vi "interface.vi"(8 "error in (no error)":errorcluster) -> (0 "error out":errorcluster)   [LabVIEW 2020]
uses:
  Control 1.ctl
  <vilib>/Utility/sysdir.llb/System Directory Type.ctl
  <vilib>/Utility/miscctls.llb/LVRowAndColumnUnsignedTypeDef.ctl
  <vilib>/Utility/config.llb/Write Key (String).vi
  <vilib>/Utility/config.llb/Write Key (Path).vi
  <vilib>/Utility/config.llb/Read Key (String).vi
  <vilib>/Utility/config.llb/Read Key (Path).vi
  _Common_Lib/UI/Window Msg/Window Msg.lvclass
  <vilib>/WebDAVClient/NI_WebDAV.lvlib
  <vilib>/Utility/config.llb/NI_LVConfig.lvlib
panel:
  in  "Delete cRIO folder(s) after download":bool
  in  "Download folder":path
  in  "Search directories":bool
  in  "cRIO IP address":string="172.22.11.2"
  in  "Open folder after download":bool
  in  "Folder path":string="/home/lvuser"
  in  "Start retrieving directories":bool
  in  "Directories list":i32[](listbox)
  # "Please select all folders that have to be retrieved from cRIO"
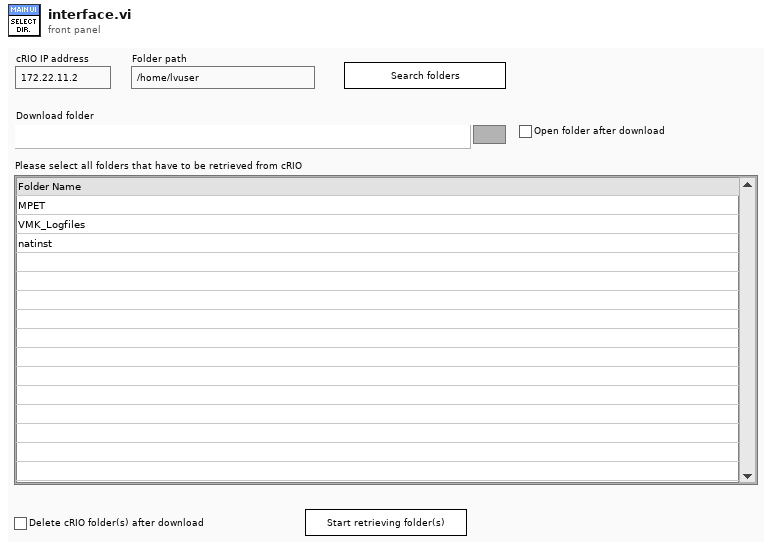
[diagram p1: front panel]
types:
  T1 = typedef "System Directory Type.ctl" = i32
  T2 = typedef "Control 1.ctl" = enum16{"READ CRIO FOLDERS", "DOWNLOAD", "IDLE", "READ SETTINGS", "ERROR", "EXIT"}
  T3 = typedef "LVRowAndColumnUnsignedTypeDef.ctl" = cluster{"Row":u32, "Column":u32}
  T4 = enum16{"INIT", "LOAD", "IDLE", "GRAPH", "ERROR", "EXIT"}
  T5 = typedef "NI_WebDAV.lvlib/SessionHandle.ctl" = refnum<k1>
  T6 = typedef "NI_WebDAV.lvlib/FileInfo.ctl" = cluster{"type":string, "size":u64, "last modification":timestamp, "display name":string, "uri":string}
  T7 = typedef "NI_LVConfig.lvlib/Config Data RefNum.ctl" = refnum<k1>
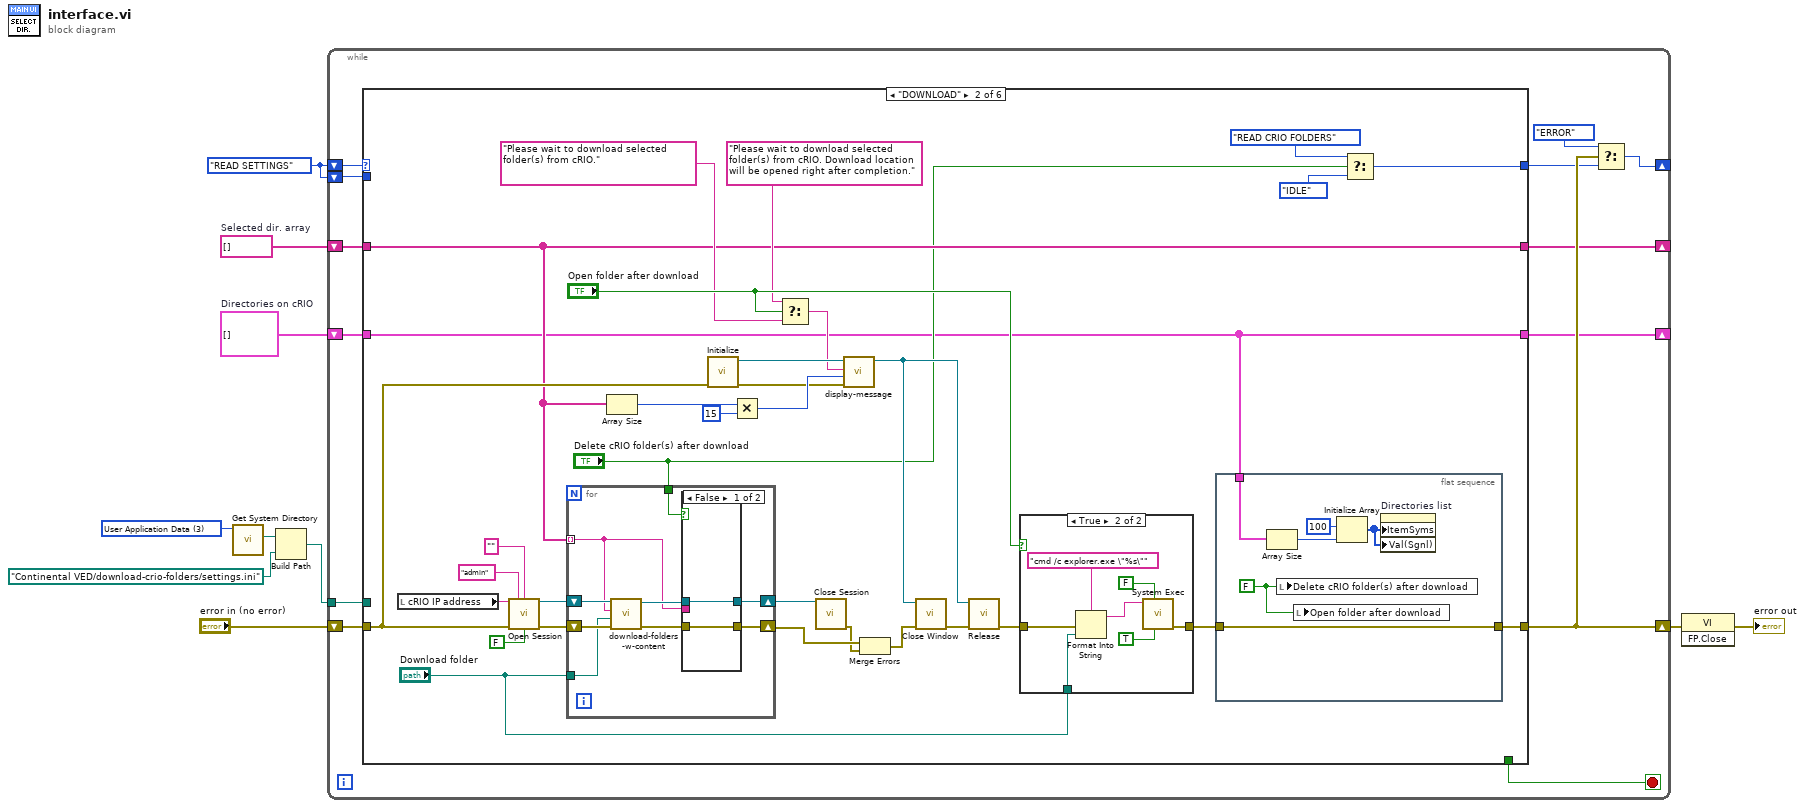
[diagram p0: block diagram]
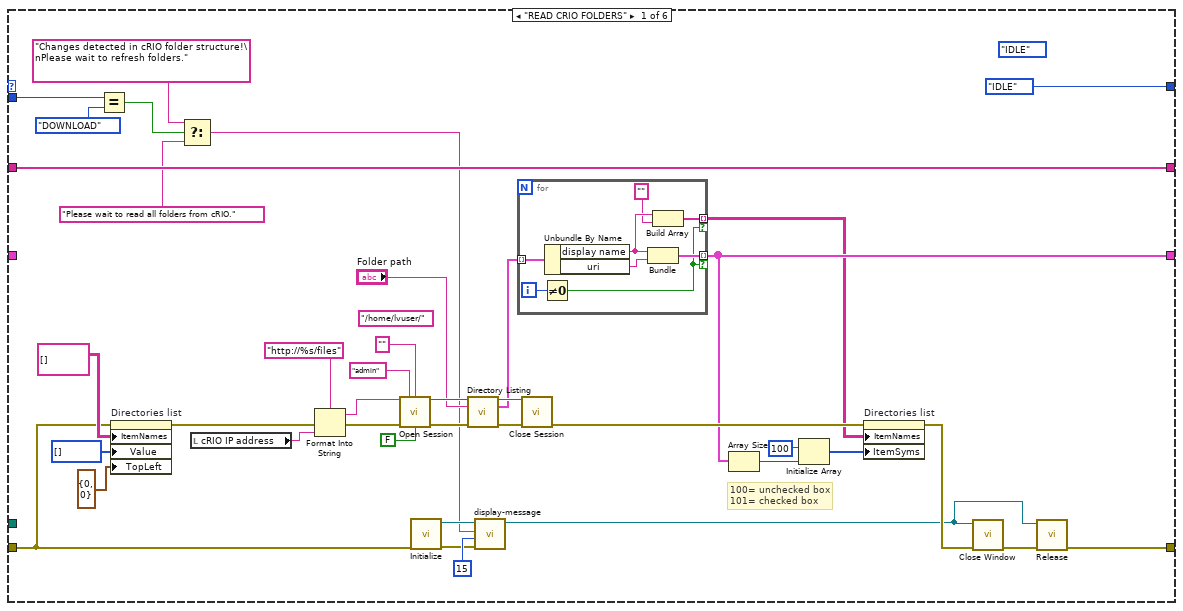
[diagram p2: hidden frame]
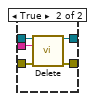
[diagram p4: hidden frame]
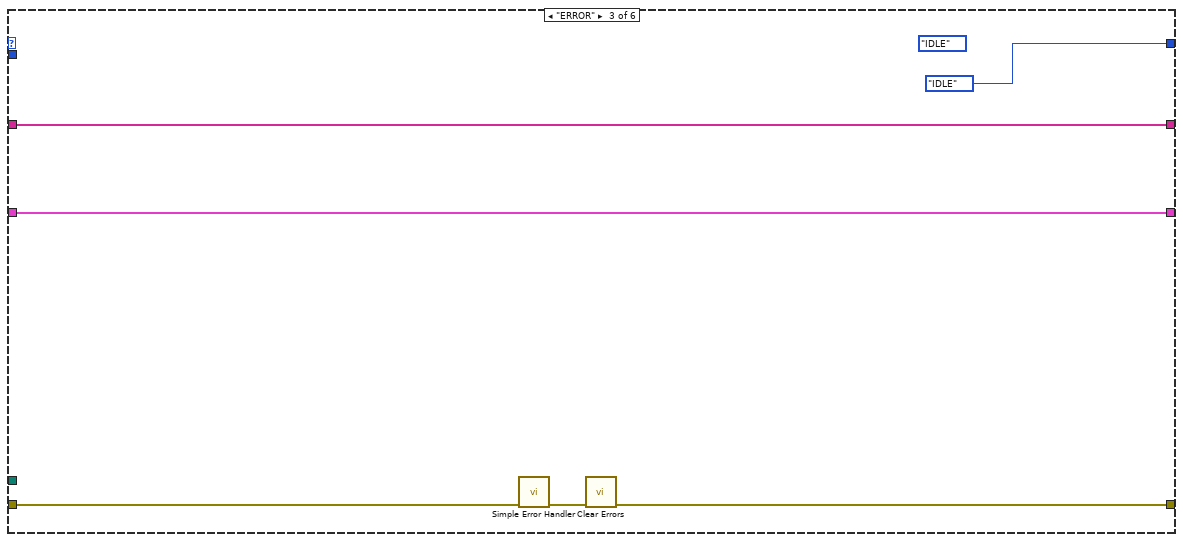
[diagram p5: hidden frame]
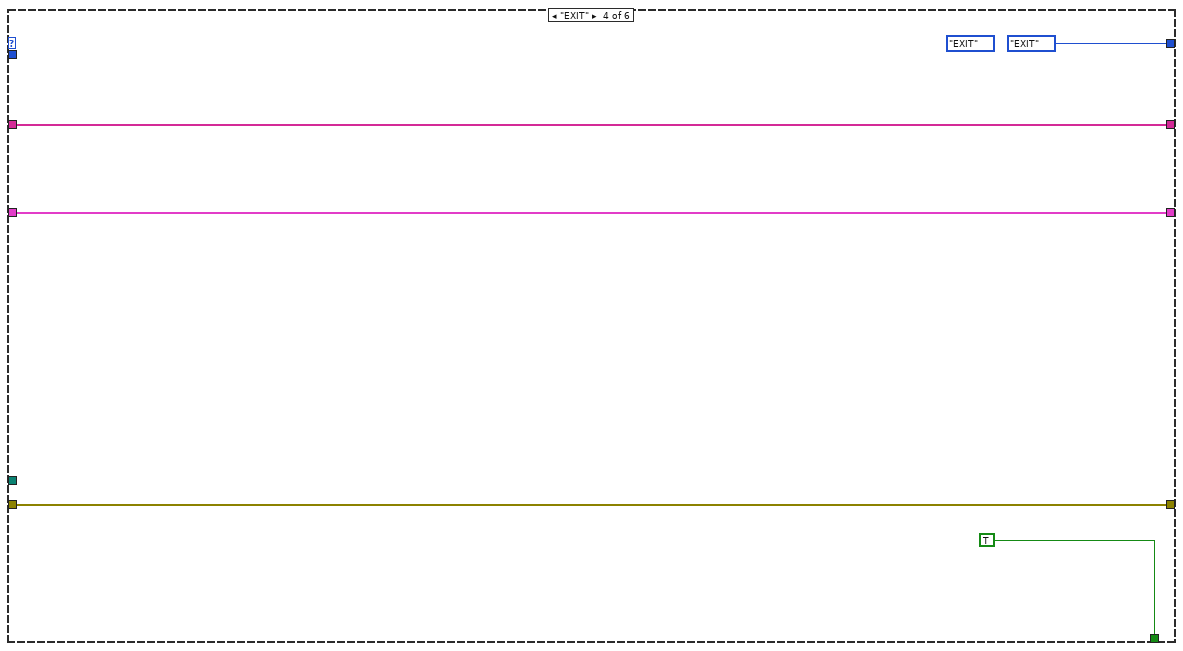
[diagram p6: hidden frame]
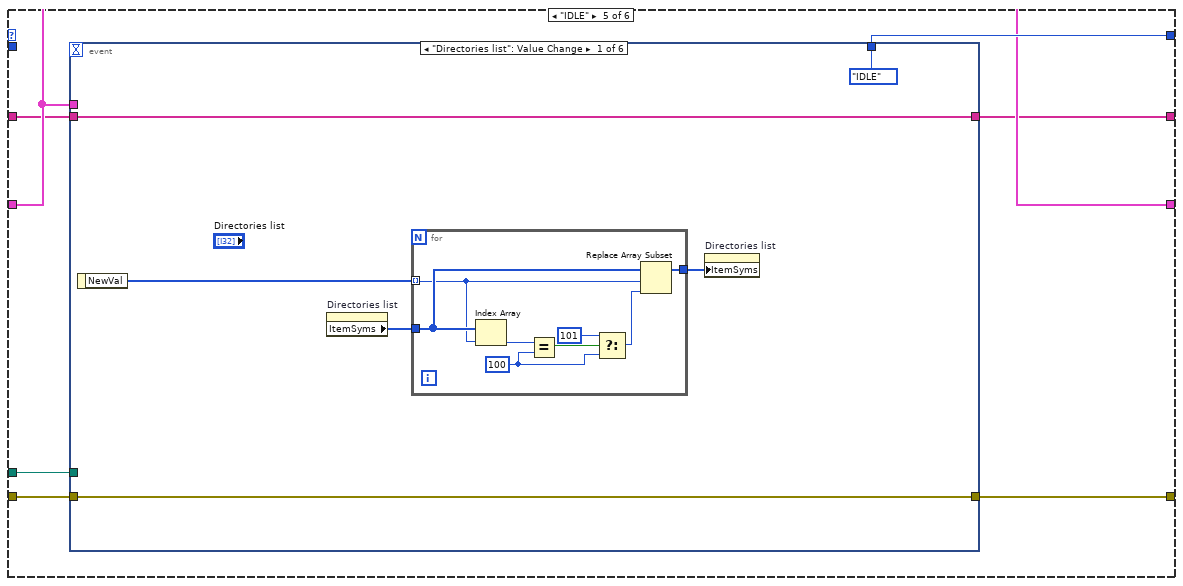
[diagram p7: hidden frame]
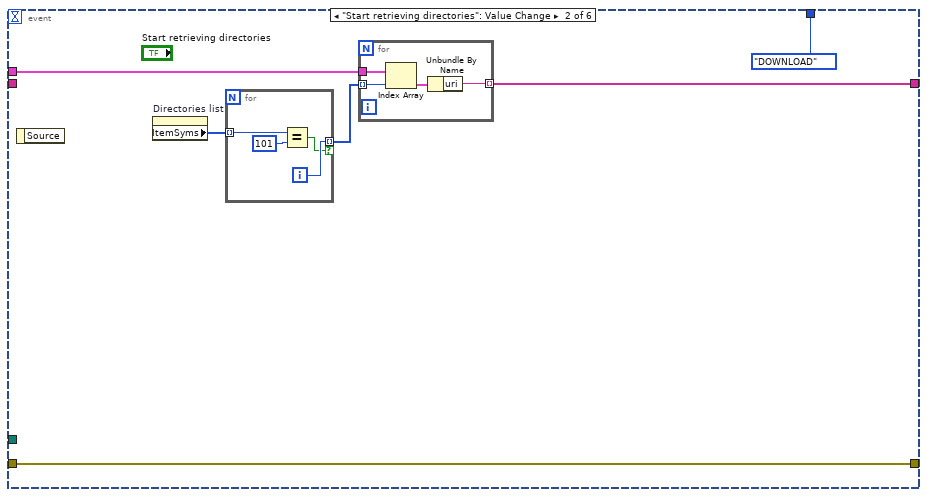
[diagram p8: hidden frame]
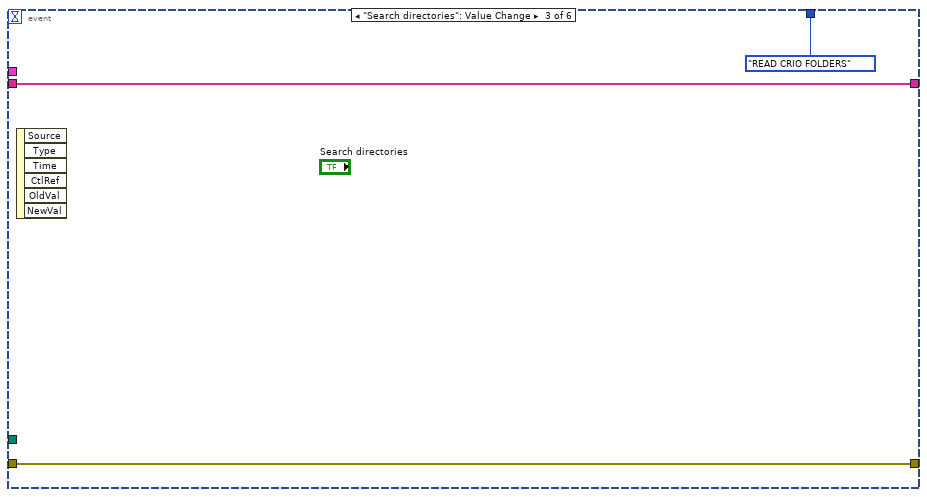
[diagram p9: hidden frame]
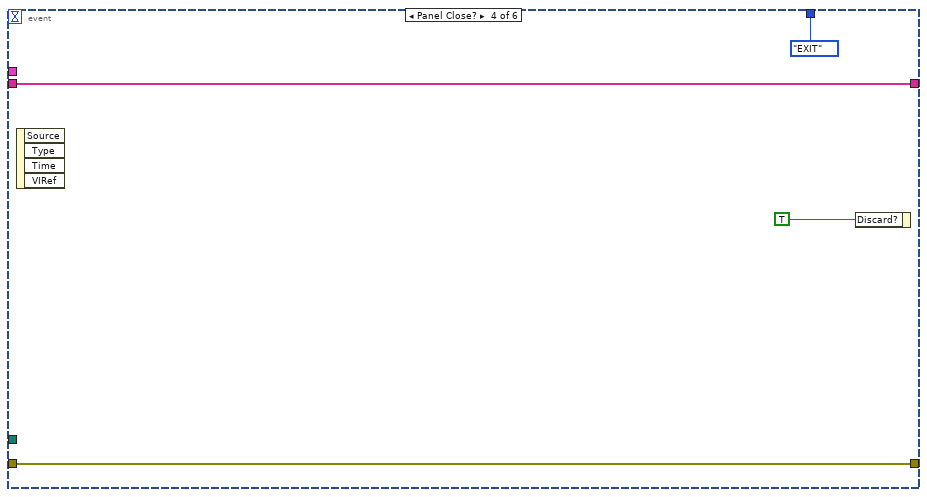
[diagram p10: hidden frame]
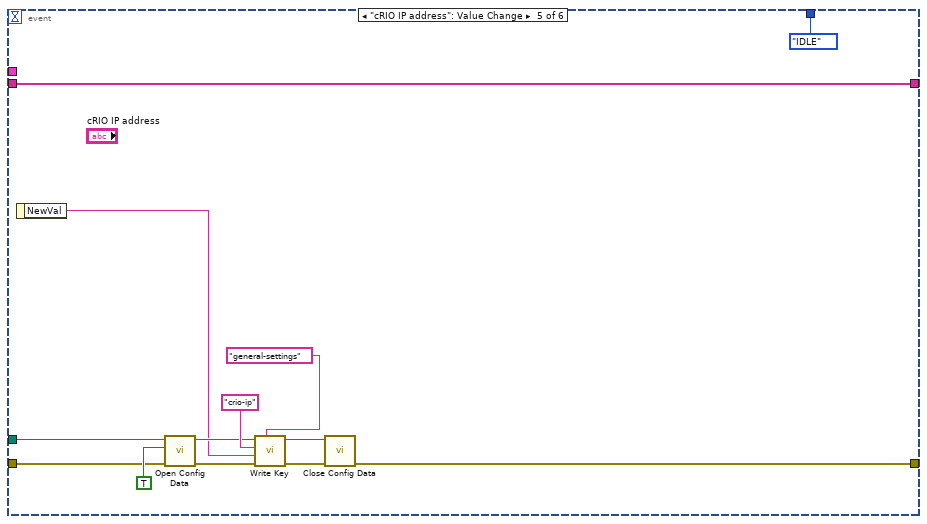
[diagram p11: hidden frame]
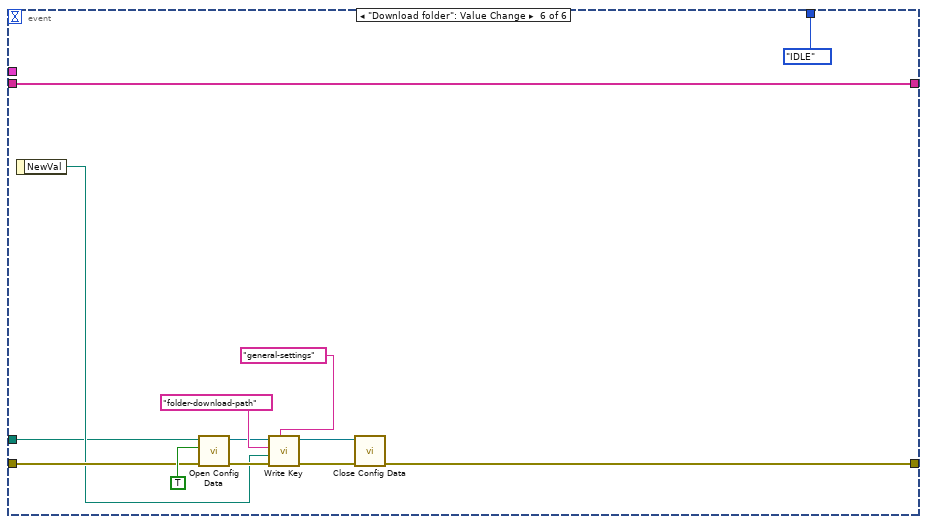
[diagram p12: hidden frame]
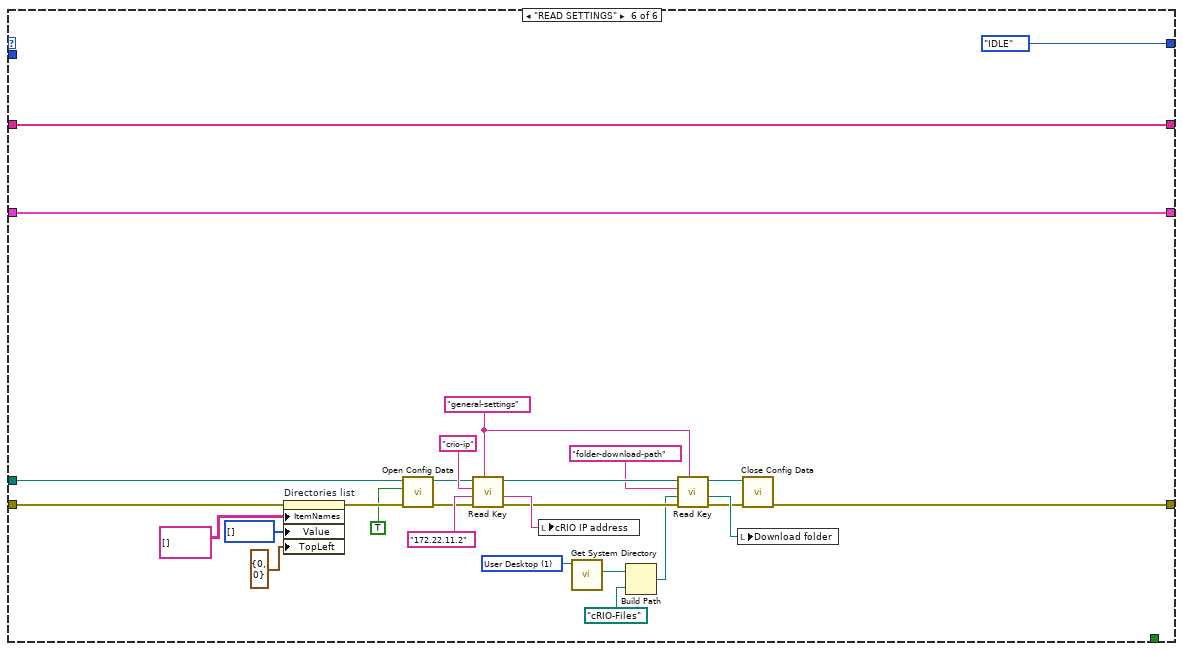
[diagram p13: hidden frame]
diagram:
  w5 = T1 3 items=["User Home"=0, "User Desktop"=1, "User Documents"=2, "User Application Data"=3, "User Preferences"=4, "User Temporary"=5, "Public Documents"=6, "Public Application Data"=7, "Public Preferences"=8, "Public Cache"=13, "System Core Libraries"=9, "System Installed Libraries"=10, "Application Files"=11, "Boot Volume Root"=12] ("system directory type")
  w1 = Control_1."READ SETTINGS" ("Motor Logger Viewer Action")
  w9 = string[] []  # Selected dir. array
  w10 = cluster{"display name":string, "uri":string}[] []  # Directories on cRIO
  n1 = call <vilib>:"Get System Directory.vi"("system directory type"=w5) -> ("system directory"=w4:path)  [unwired: 10 in]
  n2 = Build Path(base path=w4, name or relative path=path "Continental VED/download-crio-folders/settings.ini" ("configuration file path")) -> (appended path=w2:path)
  n3 = while {
    shift-right: [w20] -> w8
    shift-left: "error in (no error)" -> [w22]
    shift-right: [w18] -> _
    shift-left: w1 -> [w23]
    shift-right: [w17] -> _
    shift-left: w10 -> [w16]
    shift-right: [w15] -> _
    shift-left: w9 -> [w14]
    tunnel: w2 -> [w13]
    shift-left: w1 -> [w11]
    stop <- w21 stop-if-true
    n4 = case shown="\"DOWNLOAD\"" w23 {
      tunnel: w22 -> [w48 w93 w137 w142 w144 w214]
      tunnel: [w38 w76 w136 w142 w145 w215] -> w20
      tunnel: [_ _ _ TRUE _ _] -> w21
      tunnel: [Control_1."IDLE" ("Motor Logger Viewer Action") w72 Control_1."IDLE" ("Motor Logger Viewer Action") Control_1."EXIT" ("Motor Logger Viewer Action") w150 Control_1."IDLE" ("Motor Logger Viewer Action")] -> w19
      tunnel: [w42 w71 w135 w141 w149 w238] -> w17
      tunnel: w16 -> [_ w71 w135 w141 w149 w238]
      tunnel: [w40 w83 w134 w140 w148 w237] -> w15
      tunnel: w14 -> [w40 w83 w134 w140 w147 w237]
      tunnel: w13 -> [_ _ _ _ w146 w213]
      tunnel: w11 -> [w30 _ _ _ _ _]
      frame "READ CRIO FOLDERS" {
        (unwired) T4."IDLE" ("Motor Logger Viewer Action")
        (unwired) "/home/lvuser/" ("relative uri")
        # "100= unchecked box\n101= checked box"
        n5 = Equal?(x=w30, y=Control_1."DOWNLOAD") -> (x = y?=w28:bool)
        n6 = property on="Directories list" class="MCListbox (strict)"(error in=w48, "ItemNames"=string[][] [] ("Item Names"), "Value"=i32[] [] ("Directories list"), "TopLeft"=T3 {"Row"=0, "Column"=0} ("Top Left Visible Cell")) -> (error out=w36:errorcluster)  [unwired: 1 in, 1 out]
        n7 = Select(t="Changes detected in cRIO folder structure!\nPlease wait to refresh folders.", s=w28, f="Please wait to read all folders from cRIO." ("Message")) -> (s? t:f=w25:string)
        n8 = local read "cRIO IP address"() -> (w32:string)
        n9 = Format Into String(format string="http://%s/files", error in=w36, w32) -> (resulting string=w56:string, error out=w53:errorcluster)  [unwired: 1 in]
        n10 = call <vilib>:"Open Session.vi"("host uri prefix"=w56, "username"="admin", "password"="", "error in (no error)"=w53, "verify server?"=FALSE) -> ("session handle out"=w62:T5, "error out"=w61:errorcluster)  [unwired: 9 in]
        n11 = call "Initialize.vi"("error in (no error)"=w48) -> ("error out"=w33:errorcluster, "Window Msg out"=w52:refnum<class "Window Msg.lvclass">)  [unwired: 9 in]
        n12 = call <vilib>:"Directory Listing.vi"("session handle"=w62, "relative uri"="Folder path", "error in (no error)"=w61) -> ("session handle out"=w54:T5, "directory list"=w50:T6[], "error out"=w55:errorcluster)  [unwired: 9 in, 1 out]
        n13 = call "display-message.vi"("error in (no error)"=w33, "Time to wait (x*100ms)"=15 ("Time to wait (*500ms)"), "Message"=w25, "Window Msg in"=w52) -> ("Window Msg out"=w35:refnum<class "Window Msg.lvclass">)  [unwired: 6 in, 1 out]
        n14 = for {
          tunnel: w50 -> [w70] mode=indexing
          tunnel: [w68] -> w42 mode=indexing if=w63
          tunnel: [w64] -> w24 mode=indexing if=w63
          i -> [w67]
          n15 = Not Equal To 0?(x=w67) -> (x != 0?=w63:bool)
          n16 = Unbundle By Name(w70) -> ("display name"=w66:string, "uri"=w69:string)
          n17 = Bundle("display name"=w66, "uri"=w69) -> (w68:cluster{"display name":string, "uri":string})  [unwired: 1 in]
          n18 = Build Array(w66, "" ("display name")) -> (w64:string[])
        }
        n19 = call <vilib>:"Close Session.vi"("session handle"=w54, "error in (no error)"=w55) -> ("error out"=w45:errorcluster)  [unwired: 13 in]
        n20 = Array Size(array=w42) -> (size(s)=w43:i32)
        n21 = Initialize Array(100, w43) -> (w41:i32[])
        n22 = property on="Directories list" class="MCListbox (strict)"(error in=w45, "ItemNames"=w24, "ItemSyms"=w41) -> (error out=w39:errorcluster)  [unwired: 1 in, 1 out]
        n23 = call "Close Window.vi"("error in (no error)"=w39, "Window Msg in"=w35) -> ("error out"=w51:errorcluster)  [unwired: 9 in]
        n24 = call "Release.vi"("error in (no error)"=w51, "Window Msg in"=w35) -> ("error out"=w38:errorcluster)  [unwired: 9 in]
      }
      frame "DOWNLOAD" {
        n25 = local read "cRIO IP address"() -> (w99:string)
        n26 = call <vilib>:"Open Session.vi"("host uri prefix"=w99, "username"="admin", "password"="", "error in (no error)"=w93, "verify server?"=FALSE) -> ("session handle out"=w97:T5, "error out"=w98:errorcluster)  [unwired: 9 in]
        n27 = for {
          shift-right: [w125] -> w96
          shift-left: w98 -> [w121]
          tunnel: "Download folder" -> [w120]
          tunnel: "Delete cRIO folder(s) after download" -> [w124]
          shift-right: [w123] -> w84
          shift-left: w97 -> [w122]
          tunnel: w83 -> [w117] mode=indexing
          n28 = call "download-folders-w-content.vi"("error in"=w121, "download folder"=w120, "relative uri"=w117, "session handle in"=w122) -> ("error out"=w119:errorcluster, "session handle out"=w118:T5)  [unwired: 6 in]
          n29 = case shown="False" w124 {
            tunnel: w117 -> [_ w132]
            tunnel: w119 -> [w127 w131]
            tunnel: [w127 w130] -> w125
            tunnel: w118 -> [w126 w129]
            tunnel: [w126 w128] -> w123
            frame False {
            }
            frame True {
              n30 = call <vilib>:"Delete.vi"("session handle"=w129, "relative uri"=w132, "error in (no error)"=w131) -> ("session handle out"=w128:T5, "error out"=w130:errorcluster)  [unwired: 11 in]
            }
          }
        }
        n31 = Array Size(array=w83) -> (size(s)=w92:i32)
        n32 = call "Initialize.vi"("error in (no error)"=w93) -> ("error out"=w79:errorcluster, "Window Msg out"=w82:refnum<class "Window Msg.lvclass">)  [unwired: 9 in]
        n33 = Multiply(x=w92, y=15) -> (x*y=w80:i32)
        n34 = Select(t="Please wait to download selected folder(s) from cRIO. Download location will be opened right after completion." ("Message"), s="Open folder after download", f="Please wait to download selected folder(s) from cRIO." ("Message")) -> (s? t:f=w81:string)
        n35 = call <vilib>:"Close Session.vi"("session handle"=w84) -> ("error out"=w95:errorcluster)  [unwired: 14 in]
        n36 = call "display-message.vi"("error in (no error)"=w79, "Time to wait (x*100ms)"=w80, "Message"=w81, "Window Msg in"=w82) -> ("Window Msg out"=w78:refnum<class "Window Msg.lvclass">)  [unwired: 6 in, 1 out]
        n37 = Merge Errors(w96, w95) -> (w90:errorcluster)
        n38 = call "Close Window.vi"("error in (no error)"=w90, "Window Msg in"=w78) -> ("error out"=w94:errorcluster)  [unwired: 9 in]
        n39 = call "Release.vi"("error in (no error)"=w94, "Window Msg in"=w78) -> ("error out"=w89:errorcluster)  [unwired: 9 in]
        n40 = case shown="True" "Open folder after download" {
          tunnel: "Download folder" -> [_ w112]
          tunnel: [w109 w111] -> w77
          tunnel: w89 -> [w109 w110]
          frame False {
          }
          frame True {
            n41 = Format Into String(format string="cmd /c explorer.exe \"%s\"" ("command line"), error in=w110, w112) -> (resulting string=w115:string)  [unwired: 1 in, 1 out]
            n42 = call <vilib>:"System Exec.vi"("run minimized? (F)"=TRUE, "wait until completion? (T)"=FALSE, "command line"=w115) -> ("error out"=w111:errorcluster)  [unwired: 5 in, 3 out]
          }
        }
        n43 = flat-sequence {
          tunnel: w77 -> [w108]
          tunnel: [w108] -> w76
          tunnel: w71 -> [w104]
          frame #0 {
            w107 = FALSE ("Delete cRIO folder(s) after download")
            n44 = Array Size(array=w104) -> (size(s)=w106:i32)
            n45 = local write "Delete cRIO folder(s) after download"(w107) -> ()
            n46 = local write "Open folder after download"(w107) -> ()
            n47 = Initialize Array(100, w106) -> (w103:i32[])
            n48 = property on="Directories list" class="MCListbox (strict)"("ItemSyms"=w103, "Val(Sgnl)"=w103) -> ()  [unwired: 2 in, 2 out]
          }
        }
        n49 = Select(t=Control_1."READ CRIO FOLDERS" ("Motor Logger Viewer Action"), s="Delete cRIO folder(s) after download", f=Control_1."IDLE") -> (s? t:f=w72:T2)
      }
      frame "ERROR" {
        (unwired) T4."IDLE" ("Motor Logger Viewer Action")
        n50 = call <vilib>:"Simple Error Handler.vi"("error in (no error)"=w137) -> ("error out"=w138:errorcluster)  [unwired: 4 in, 4 out]
        n51 = call <vilib>:"Clear Errors.vi"("error in (no error)"=w138) -> ("error out"=w136:errorcluster)  [unwired: 5 in, 1 out]
      }
      frame "EXIT" {
        (unwired) T4."EXIT" ("Motor Logger Viewer Action")
      }
      frame "IDLE" {
        n52 = event shown="[0] \"Directories list\": Value Change" {
          selector: _ -> [_ _ _ _ _ _]
          dyn-events: _ -> [_ _ _ _ _ _]
          timeout: _ -> [_ _ _ _ _ _]
          tunnel: [Control_1."IDLE" ("Motor Logger Viewer Action") Control_1."DOWNLOAD" ("Motor Logger Viewer Action") Control_1."READ CRIO FOLDERS" ("Motor Logger Viewer Action") Control_1."EXIT" ("Motor Logger Viewer Action") Control_1."IDLE" ("Motor Logger Viewer Action") Control_1."IDLE" ("Motor Logger Viewer Action")] -> w150
          tunnel: w149 -> [_ w169 _ _ _ _]
          tunnel: [w153 w167 w181 w184 w198 w211] -> w148
          tunnel: w147 -> [w153 _ w181 w184 w198 w211]
          tunnel: w146 -> [_ _ _ _ w193 w200]
          tunnel: w144 -> [w152 w166 w180 w183 w192 w203]
          tunnel: [w152 w166 w180 w183 w191 w202] -> w145
          event "Directories list": Value Change {
            n53 = event-data() -> ("NewVal"=w156:i32[])  [unwired: 1 in]
            n54 = property on="Directories list" class="MCListbox (strict)"() -> ("ItemSyms"=w155:i32[])  [unwired: 2 in, 2 out]
            n55 = for {
              tunnel: w156 -> [w158] mode=indexing
              tunnel: w155 -> [w160]
              tunnel: [w157] -> w154
              w162 = 100 ("y")
              n56 = Index Array(array=w160, index=w158) -> (element=w164:i32)
              n57 = Equal?(x=w164, y=w162) -> (x = y?=w163:bool)
              n58 = Select(t=101, s=w163, f=w162) -> (s? t:f=w159:i32)
              n59 = Replace Array Subset(array=w160, new element=w159, index=w158) -> (w157:i32[])
            }
            n60 = property on="Directories list" class="MCListbox (strict)"("ItemSyms"=w154) -> ()  [unwired: 2 in, 2 out]
          }
          event "Start retrieving directories": Value Change {
            n61 = event-data() -> ()  [unwired: 1 in, 1 out]
            n62 = property on="Directories list" class="MCListbox (strict)"() -> ("ItemSyms"=w170:i32[])  [unwired: 2 in, 2 out]
            n63 = for {
              tunnel: w170 -> [w178] mode=indexing
              tunnel: [w176] -> w168 mode=indexing if=w175
              i -> [w176]
              n64 = Equal?(x=w178, y=101) -> (x = y?=w175:bool)
            }
            n65 = for {
              tunnel: w169 -> [w174]
              tunnel: w168 -> [w173] mode=indexing
              tunnel: [w171] -> w167 mode=indexing
              n66 = Index Array(array=w174, index=w173) -> (element=w172:cluster{"display name":string, "uri":string})
              n67 = Unbundle By Name(w172) -> ("uri"=w171:string)
            }
          }
          event "Search directories": Value Change {
            n68 = event-data() -> ()  [unwired: 1 in, 6 out]
          }
          event Panel Close? {
            n69 = event-data() -> ()  [unwired: 1 in, 4 out]
            n70 = event-data("Discard?"=TRUE) -> ()  [unwired: 1 in, 1 out]
          }
          event "cRIO IP address": Value Change {
            n71 = event-data() -> ("NewVal"=w187:string)  [unwired: 1 in]
            n72 = call <vilib>:"Open Config Data.vi"("error in (no error)"=w192, "create file if necessary (T)"=TRUE, "configuration file path"=w193) -> ("error out"=w196:errorcluster, "refnum"=w195:T7)  [unwired: 6 in, 1 out]
            n73 = call-poly <vilib>:"Write Key.vi"("section"="general-settings", "error in (no error)"=w196, "value"=w187, "key"="crio-ip", "refnum"=w195) -> ("error out"=w189:errorcluster, "refnum out"=w190:T7)  [unwired: 4 in, 1 out]
            n74 = call <vilib>:"Close Config Data.vi"("error in (no error)"=w189, "refnum"=w190) -> ("error out"=w191:errorcluster)  [unwired: 8 in, 1 out]
          }
          event "Download folder": Value Change {
            n75 = event-data() -> ("NewVal"=w201:path)  [unwired: 1 in]
            n76 = call <vilib>:"Open Config Data.vi"("error in (no error)"=w203, "create file if necessary (T)"=TRUE, "configuration file path"=w200) -> ("error out"=w209:errorcluster, "refnum"=w208:T7)  [unwired: 6 in, 1 out]
            n77 = call-poly <vilib>:"Write Key.vi"("section"="general-settings", "error in (no error)"=w209, "value"=w201, "key"="folder-download-path", "refnum"=w208) -> ("error out"=w205:errorcluster, "refnum out"=w206:T7)  [unwired: 4 in, 1 out]
            n78 = call <vilib>:"Close Config Data.vi"("error in (no error)"=w205, "refnum"=w206) -> ("error out"=w202:errorcluster)  [unwired: 8 in, 1 out]
          }
        }
      }
      frame "READ SETTINGS" {
        w233 = "general-settings" ("section")
        w216 = T1 1 items=["User Home"=0, "User Desktop"=1, "User Documents"=2, "User Application Data"=3, "User Preferences"=4, "User Temporary"=5, "Public Documents"=6, "Public Application Data"=7, "Public Preferences"=8, "Public Cache"=13, "System Core Libraries"=9, "System Installed Libraries"=10, "Application Files"=11, "Boot Volume Root"=12] ("system directory type")
        n79 = property on="Directories list" class="MCListbox (strict)"(error in=w214, "ItemNames"=string[][] [] ("Item Names"), "Value"=i32[] [] ("Directories list"), "TopLeft"=T3 {"Row"=0, "Column"=0} ("Top Left Visible Cell")) -> (error out=w231:errorcluster)  [unwired: 1 in, 1 out]
        n80 = call <vilib>:"Open Config Data.vi"("error in (no error)"=w231, "create file if necessary (T)"=TRUE, "configuration file path"=w213) -> ("error out"=w228:errorcluster, "refnum"=w227:T7)  [unwired: 6 in, 1 out]
        n81 = call-poly <vilib>:"Read Key.vi"("section"=w233, "error in (no error)"=w228, "default value"="172.22.11.2", "key"="crio-ip", "refnum"=w227) -> ("error out"=w229:errorcluster, "value"=w232:string, "refnum out"=w230:T7)  [unwired: 3 in, 1 out]
        n82 = local write "cRIO IP address"(w232) -> ()
        n83 = call <vilib>:"Get System Directory.vi"("system directory type"=w216) -> ("system directory"=w217:path)  [unwired: 10 in]
        n84 = Build Path(base path=w217, name or relative path=path "cRIO-Files" ("base path")) -> (appended path=w222:path)
        n85 = call-poly <vilib>:"Read Key.vi"("section"=w233, "error in (no error)"=w229, "default value"=w222, "key"="folder-download-path", "refnum"=w230) -> ("error out"=w224:errorcluster, "value"=w235:path, "refnum out"=w225:T7)  [unwired: 3 in, 1 out]
        n86 = local write "Download folder"(w235) -> ()
        n87 = call <vilib>:"Close Config Data.vi"("error in (no error)"=w224, "refnum"=w225) -> ("error out"=w215:errorcluster)  [unwired: 8 in, 1 out]
      }
    }
    n88 = Select(t=Control_1."ERROR" ("Motor Logger Viewer Action"), s=w20, f=w19) -> (s? t:f=w18:T2)
  }
  n89 = invoke class="VI" method="FP.Close"(error in=w8) -> (error out=→"error out":errorcluster)  [unwired: 2 in, 2 out]
